vi "CM-Save Display Settings.vi"(0 "configuration file path":path=path "C:/PXI Connections.txt", 5 "Breakout box type":enum32{"BNC-2090", "BNC-2110"}(radio), 9 "Hide unused":bool, 11 "error in (no error)":errorcluster) -> (4 "file path":path, 15 "error out":errorcluster)   [LabVIEW 2015]
uses:
  <vilib>/Utility/config.llb/Write Key (Boolean).vi
  <vilib>/Utility/config.llb/NI_LVConfig.lvlib
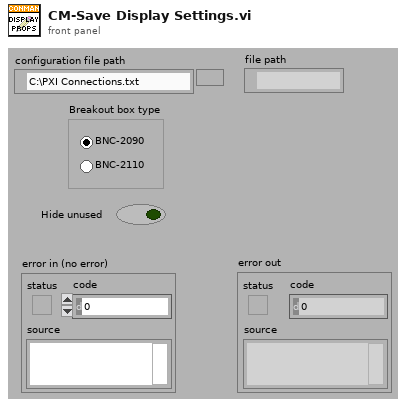
[diagram p1: front panel]
types:
  T1 = typedef "NI_LVConfig.lvlib/Config Data RefNum.ctl" = refnum<k1>
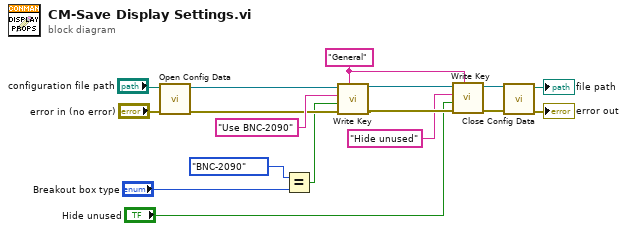
[diagram p0: block diagram]
diagram:
  w14 = "General" ("section")
  n1 = call <vilib>:"Open Config Data.vi"("error in (no error)"="error in (no error)", "configuration file path"="configuration file path") -> ("error out"=w5:errorcluster, "refnum"=w6:T1)  [unwired: 7 in, 1 out]
  n2 = Equal?(x=enum32{"BNC-2090", "BNC-2110"}."BNC-2090" ("y"), y="Breakout box type") -> (x = y?=w2:bool)
  n3 = call-poly <vilib>:"Write Key.vi"("section"=w14, "error in (no error)"=w5, "value"=w2, "key"="Use BNC-2090", "refnum"=w6) -> ("error out"=w13:errorcluster, "refnum out"=w12:T1)  [unwired: 4 in, 1 out]
  n4 = call-poly <vilib>:"Write Key.vi"("section"=w14, "error in (no error)"=w13, "value"="Hide unused", "key"="Hide unused", "refnum"=w12) -> ("error out"=w8:errorcluster, "refnum out"=w7:T1)  [unwired: 4 in, 1 out]
  n5 = call <vilib>:"Close Config Data.vi"("error in (no error)"=w8, "refnum"=w7) -> ("error out"=→"error out":errorcluster, "file path"=→"file path":path)  [unwired: 8 in]
